vi "Get Type.vi"(8 "error in (no error)":errorcluster, 11 "Logic Circuit in":refnum<class "Logic Circuit.lvclass">) -> (0 "error out":errorcluster, 2 "Item Type":T1, 3 "Logic Circuit out":refnum<class "Logic Circuit.lvclass">)   [LabVIEW 2020, in "Logic Circuit.lvclass"]
uses:
  Logic Circuit.lvclass
  Item/Item Type.ctl
  Item/Item.lvclass
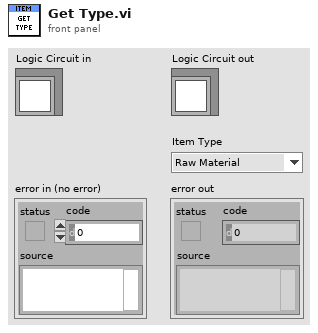
[diagram p1: front panel]
types:
  T1 = typedef "Item.lvclass/Item Type.ctl" = enum16{"Raw Material", "Component", "Module", "Product"}
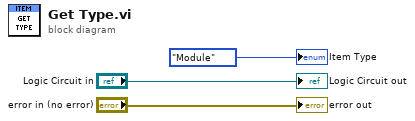
[diagram p0: block diagram]
diagram:
  "error out" <- "error in (no error)"
  "Logic Circuit out" <- "Logic Circuit in"
  "Item Type" <- Item_Type."Module" ("Item Type")
